vi "Parse Data JSON.vi"(8 "error in (no error)":errorcluster, 10 "Data JSON":string, 11 "Response in":refnum<class "Response.lvclass">) -> (0 "error out":errorcluster, 1 "Replaced?":bool, 2 "Typed Message":refnum<class "Response.lvclass">, 3 "Response out":refnum<class "Response.lvclass">)   [LabVIEW 2022 SP3, in "obs-websocket-lv.lvlib" / "Response.lvclass"]
uses:
  Response.lvclass
  Response.lvclass/Response.ctl
  <vilib>/IlluminatedG/lv-web-crypto/lv-json/JSON/JSON.lvlib
  obs-websocket-lv.lvlib
  C:/dev/illuminatedg/obs-websocket-lv/obs-websocket-lv/Server Message/Server Message.lvclass
  C:/dev/illuminatedg/obs-websocket-lv/obs-websocket-lv/Message/Message.lvclass
  C:/dev/illuminatedg/obs-websocket-lv/obs-websocket-lv/Response/Response.lvclass
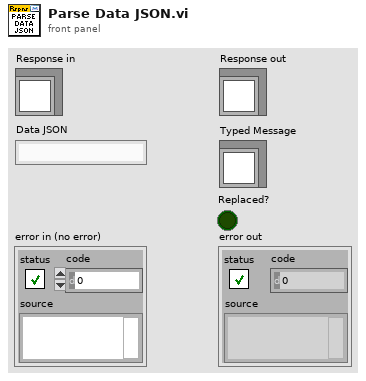
[diagram p1: front panel]
types:
  T1 = typedef "JSON.lvlib/JSON Item Type.ctl" = enum16{"unknown", "null", "Array", "Object", "String", "Number", "Boolean"}
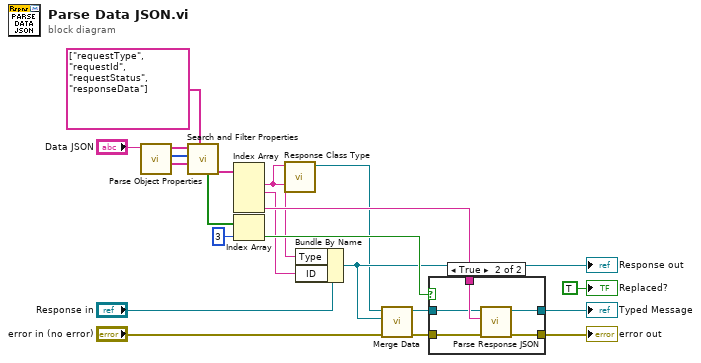
[diagram p0: block diagram]
diagram:
  n1 = call <vilib>:"Parse Object Properties.vi"("JSON String"="Data JSON") -> ("Values"=w18:string[], "Item Types"=w19:T1[], "Keys"=w20:string[])  [unwired: 7 in, 1 out]
  n2 = call <vilib>:"Search and Filter Properties.vi"("Search Keys"=string[] ["requestType", "requestId", "requestStatus", "responseData"], "Values In"=w18, "Types In"=w19, "Keys In"=w20) -> ("Filtered Values"=w16:string[], "Item Found"=w15:bool[])  [unwired: 2 in, 4 out]
  n3 = Index Array(array=w16) -> (element #1=w3:string, element #2=w1:string, element #4=w13:string)  [unwired: 4 in, 1 out]
  n4 = Index Array(array=w15, index=3) -> (element=w9:bool)
  n5 = call "Response Class Type.vi"("Type"=w3) -> ("Class"=w2:refnum<class "Response.lvclass">)  [unwired: 10 in]
  n6 = Bundle By Name(cluster="Response in", "Type"=w3, "ID"=w1) -> (w6:refnum<class "Response.lvclass">)
  "Response out" <- w6
  n7 = call-dynamic "Merge Data.vi"("error in (no error)"="error in (no error)", "From"=w6, "Typed Response in"=w2) -> ("error out"=w8:errorcluster, "Typed Response out"=w10:refnum<class "Response.lvclass">)  [unwired: 7 in]
  n8 = case shown="True" w9 {
    tunnel: w13 -> [_ w28]
    tunnel: w10 -> [w23 w27]
    tunnel: [w23 w26] -> w5
    tunnel: w8 -> [w22 w25]
    tunnel: [w22 w24] -> w7
    frame False {
    }
    frame True {
      n9 = call-dynamic "Parse Response JSON.vi"("error in (no error)"=w25, "Response JSON"=w28, "Response in"=w27) -> ("error out"=w24:errorcluster, "Response out"=w26:refnum<class "Response.lvclass">)  [unwired: 7 in]
    }
  }
  "error out" <- w7
  "Typed Message" <- w5
  "Replaced?" <- TRUE ("Replaced?")
